vi "TestPVCam_DiskStreaming.vi"(8 "error in":errorcluster, 10 "Exposure time [ms]":T7=25) -> (0 "error out":errorcluster)   [LabVIEW 2023, in "Photometrics Camera.lvlib"]
uses:
  Photometrics Camera.lvlib
  <userlib>/TPM LabVIEW adapter/SDK/Controls/Camera Description.ctl
  <userlib>/TPM LabVIEW adapter/SDK/Controls/Exposure Time.ctl
  <userlib>/TPM LabVIEW adapter/SDK/Controls/Frames To Capture.ctl
  <userlib>/TPM LabVIEW adapter/SDK/Controls/Frames Captured.ctl
  <userlib>/TPM LabVIEW adapter/SDK/Controls/Disk Streaming Options.ctl
  <userlib>/TPM LabVIEW adapter/SDK/Controls/Disk Streaming File Name.ctl
  <userlib>/TPM LabVIEW adapter/SDK/Controls/Disk Streaming File Size.ctl
  <userlib>/TPM LabVIEW adapter/PVCAM/PVCAM.lvclass
  <userlib>/TPM LabVIEW adapter/SDK/Controls/All Params IDs.ctl
  <userlib>/TPM LabVIEW adapter/SDK/Controls/Acquisition Mode.ctl
  <userlib>/TPM LabVIEW adapter/SDK/Controls/Region Index.ctl
  <userlib>/TPM LabVIEW adapter/SDK/Controls/Buffer Size.ctl
  <userlib>/TPM LabVIEW adapter/Camera/Camera.lvclass
panel:
  in  "Disk Streaming Options":T1={"Disk Streaming File Name"="test", "Path"=path "E:/", "File Format"=enum."RAW", "File Size"=1000000000000, "Big TIFF required"=FALSE}
  out "Frames Captured":T4
  out "Image":T5(plugin-control)
  in  "Frames To Capture":T6=1000
  out "Disk Streaming Failed":bool
  out "Disk Streaming Dropped Frames":u64
  out "FPS":dbl
  out "Disk Streaming Queue Count":u32
  out "Camera Description":T8
  out "Number of cameras":u32
  out "Camera 0 Name":string
  out "output array":u16[][](array[numeric])
  in  "STOP":bool
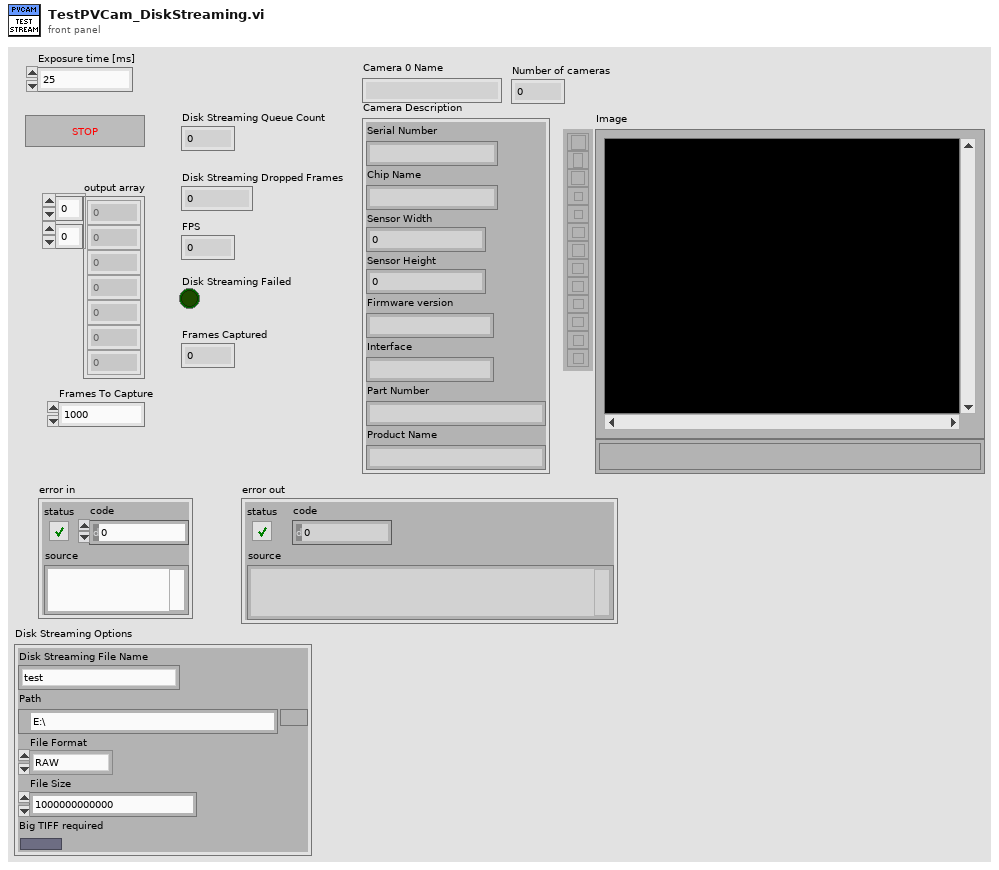
[diagram p1: front panel]
types:
  T1 = typedef "Disk Streaming Options.ctl" = cluster{"Disk Streaming File Name":T2, "Path":path, "File Format":enum32{"RAW", "TIFF"}, "File Size":T3, "Big TIFF required":bool}
  T2 = typedef "Disk Streaming File Name.ctl" = string
  T3 = typedef "Disk Streaming File Size.ctl" = u64
  T4 = typedef "Frames Captured.ctl" = u64
  T5 = typedef "IMAQ Image.ctl" = refnum<image>
  T6 = typedef "Frames To Capture.ctl" = u32
  T7 = typedef "Exposure Time.ctl" = u32
  T8 = typedef "Camera Description.ctl" = cluster{"Serial Number":string, "Chip Name":string, "Sensor Width":u32, "Sensor Height":u32, "Firmware version":string, "Interface":string, "Part Number":string, "Product Name":string}
  T9 = typedef "Buffer Size.ctl" = u32
  T10 = typedef "Region Index.ctl" = i32
  T11 = typedef "Acquisition Mode.ctl" = enum16{"Sequence", "Live"}
  T12 = typedef "All Params IDs.ctl" = i32
  T13 = typedef "Camera Regions.ctl" = T14[]
  T14 = typedef "Region.ctl" = cluster{"Origin X":u16, "Origin Y":u16, "Width":u16, "Height":u16}
  T15 = typedef "Acquisition Status.ctl" = enum32{"Idle", "Starting", "Acquiring", "Stopping"}
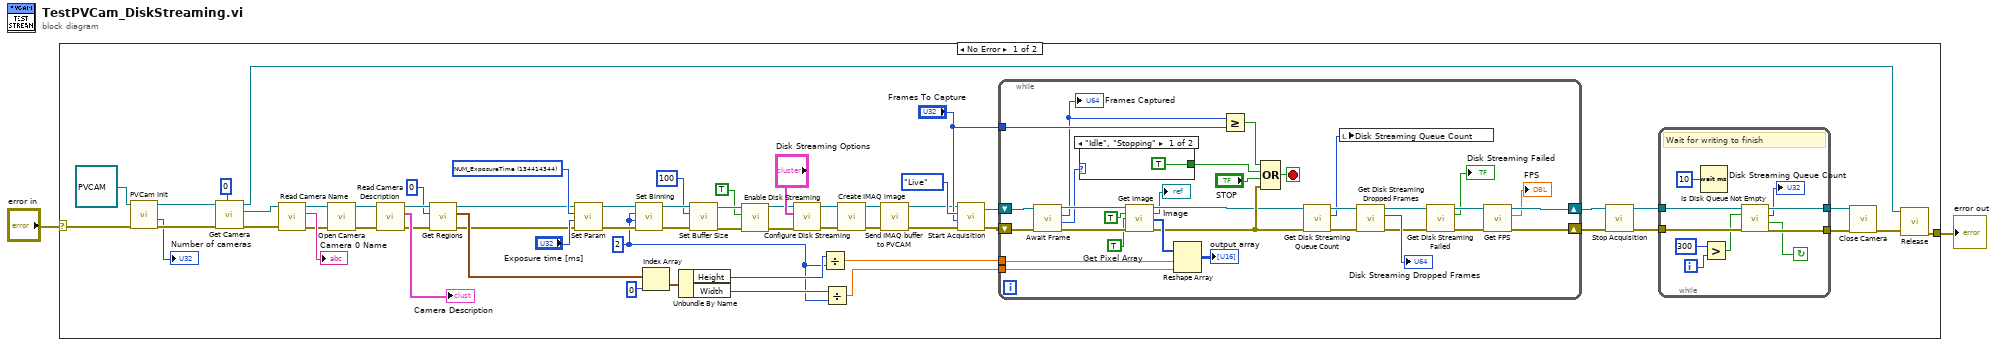
[diagram p0: block diagram]
diagram:
  n1 = case shown="No Error" "error in" {
    selector: "error in" -> [w30 w105]
    tunnel: [w41 w105] -> w2
    frame No Error {
      w8 = u16 2 ("Binning X")
      w47 = T12 134414344 items=["BOOL_BofEofClr"=184745991, "BOOL_CentroidsEnabled"=184746154, "BOOL_CircBuffer"=184746283, "BOOL_FrameCapable"=184680957, "BOOL_GainMultEnable"=184680989, "BOOL_MetadataEnabled"=184746152, "BOOL_MetadataResetTimestamp"=184746160, "BOOL_ScanDirectionReset"=184746236, "BOOL_SmartStreamModeEnabled"=184681148, "ENUM_BinningPar"=151191718, "ENUM_BinningSer"=151191717, "ENUM_BofEofEnable"=151191557, "ENUM_CamInterfaceMode"=150994955, "ENUM_CamInterfaceType"=150994954, "ENUM_CentroidsBgCount"=151191726, "ENUM_CentroidsMode"=151191725, "ENUM_ClearMode"=151126539, "ENUM_ColorMode"=151126520, "ENUM_CoolingMode"=151126230, "ENUM_ExpRes"=151191554, "ENUM_ExposeOutMode"=151126576, "ENUM_ExposureMode"=151126551, "ENUM_FanSpeedSetpoint"=151126726, "ENUM_FrameFlip"=151126273, "ENUM_FrameRotate"=151126272, "ENUM_ImageCompression"=151126265, "ENUM_ImageFormat"=151126264, "ENUM_IoDirection"=151126545, "ENUM_IoType"=151126544, "ENUM_MppCapable"=151126240, "ENUM_PMode"=151126540, "ENUM_ReadoutPort"=151126263, "ENUM_ScanDirection"=151191803, "ENUM_ScanMode"=151191802, "ENUM_ShtrOpenMode"=151126537, "ENUM_ShtrStatus"=151126538, "ENUM_TrigTabSignal"=151191732, "NUM_ActualGain"=100794912, "NUM_AdcOffset"=16908483, "NUM_BitDepth"=16908799, "NUM_BofEofCount"=117637126, "NUM_CamFwVersion"=100794900, "NUM_CentroidsCount"=100860076, "NUM_CentroidsRadius"=100860075, "NUM_CentroidsThreshold"=117637295, "NUM_ClearCycles"=100794465, "NUM_ClearingTime"=268566708, "NUM_DdInfoLength"=16777217, "NUM_DdRetries"=100663299, "NUM_DdTimeout"=100663300, "NUM_DdVersion"=100663298, "NUM_ExpResIndex"=100859908, "NUM_ExpTime"=100859905, "NUM_ExposureTime"=134414344, "NUM_FrameBufferSize"=134414636, "NUM_FwellCapacity"=117572090, "NUM_GainIndex"=16908800, "NUM_GainMultFactor"=100794905, "NUM_IoAddr"=100794895, "NUM_IoBitDepth"=100794899, "NUM_IoState"=67240466, "NUM_LastMuxedSignal"=84082869, "NUM_ParSize"=100794425, "NUM_PciFwVersion"=100794902, "NUM_PixParDist"=100794868, "NUM_PixParSize"=100794431, "NUM_PixSerDist"=100794869, "NUM_PixSerSize"=100794430, "NUM_PixTime"=100794884, "NUM_PostTriggerDelay"=268566709, "NUM_Postmask"=100794422, "NUM_Postscan"=100794424, "NUM_PreTriggerDelay"=268566710, "NUM_PreampDelay"=100794870, "NUM_PreampOffControl"=117572091, "NUM_Premask"=100794421, "NUM_Prescan"=100794423, "NUM_ReadoutTime"=67240115, "NUM_RoiCount"=100860073, "NUM_SP_PpIndex"=16908831, "NUM_SP_PpParamIndex"=16908833, "NUM_ScanLineDelay"=100860157, "NUM_ScanLineTime"=268632318, "NUM_ScanWidth"=100860159, "NUM_SerSize"=100794426, "NUM_ShtrCloseDelay"=100794887, "NUM_ShtrOpenDelay"=100794888, "NUM_SmartStreamMode"=100795069, "NUM_SpdtabIndex"=16908801, "NUM_SummingWell"=184680953, "NUM_Temp"=16908813, "NUM_TempSetpoint"=16908814, "PP_PpFeatId"=100794917, "PP_PpParam"=117572131, "PP_PpParamId"=100794918, "PP_ReadNoise"=100794916, "SS_SmartStreamDlyParams"=235012799, "SS_SmartStreamModeExpParams"=235012798, "STR_CamSystemsInfo"=218235416, "STR_CameraPartNumber"=218235013, "STR_ChipName"=218235009, "STR_DdInfo"=218103813, "STR_GainName"=218235394, "STR_HeadSerNumAlpha"=218235413, "STR_PpFeatName"=218235422, "STR_PpParamName"=218235426, "STR_ProductName"=218235012, "STR_SystemName"=218235010, "STR_VendorName"=218235011] ("PVCAM Param IDs")
      n2 = call <userlib>:"PVCam Init.vi"("error in (no error)"=w30, "PVCAM In"=refnum<class "PVCAM.lvclass"> refnum ("PVCAM.lvclass")) -> ("error out"=w58:errorcluster, "Number of cameras"=→"Number of cameras":u32, "PVCAM Out"=w60:refnum<class "PVCAM.lvclass">)  [unwired: 6 in, 1 out]
      n3 = call <userlib>:"Get Camera.vi"("Camera Index"=u32 0 ("Camera Index (0)"), "error in (no error)"=w58, "PVCAM In"=w60) -> ("error out"=w55:errorcluster, "Camera.lvclass"=w57:refnum<class "Camera.lvclass">, "PVCAM Out"=w61:refnum<class "PVCAM.lvclass">)  [unwired: 6 in]
      n4 = call <userlib>:"Read Camera Name.vi"("error in (no error)"=w55, "Camera in"=w57) -> ("error out"=w53:errorcluster, "Camera Name"=→"Camera 0 Name":string, "Camera out"=w54:refnum<class "Camera.lvclass">)  [unwired: 7 in]
      n5 = call <userlib>:"Open Camera.vi"("error in (no error)"=w53, "Camera in"=w54) -> ("error out"=w50:errorcluster, "Camera out"=w49:refnum<class "Camera.lvclass">)  [unwired: 8 in]
      n6 = call-dynamic "Read Camera Description.vi"("error in (no error)"=w50, "Camera in"=w49) -> ("error out"=w37:errorcluster, "Camera Description"=→"Camera Description":T8, "Camera out"=w38:refnum<class "Camera.lvclass">)  [unwired: 7 in]
      n7 = call <userlib>:"Get Regions.vi"("error in (no error)"=w37, "Region Index"=T10 0, "Camera in"=w38) -> ("error out"=w19:errorcluster, "Camera Regions"=w33:T13, "Camera out"=w20:refnum<class "Camera.lvclass">)  [unwired: 6 in]
      n8 = call <userlib>:"Set Param.vi"("error in (no error)"=w19, "Parameter value"="Exposure time [ms]", "PVCAM Param IDs"=w47, "Camera In"=w20) -> ("error out"=w45:errorcluster, "Camera Out"=w44:refnum<class "Camera.lvclass">)  [unwired: 6 in]
      n9 = call <userlib>:"Set Binning.vi"("error in (no error)"=w45, "Binning Y"=w8, "Binning X"=w8, "Camera in"=w44) -> ("error out"=w24:errorcluster, "Camera out"=w23:refnum<class "Camera.lvclass">)  [unwired: 6 in]
      n10 = Index Array(array=w33, index=0) -> (element=w35:T14)
      n11 = Unbundle By Name(w35) -> ("Height"=w11:u16, "Width"=w9:u16)
      n12 = call <userlib>:"Set Buffer Size.vi"("error in (no error)"=w24, "Buffer Size Frames"=T9 100, "Camera in"=w23) -> ("error out"=w6:errorcluster, "Camera out"=w7:refnum<class "Camera.lvclass">)  [unwired: 7 in]
      n13 = call <userlib>:"Enable Disk Streaming.vi"("error in (no error)"=w6, "Enable/Disable streaming"=TRUE, "Camera in"=w7) -> ("error out"=w5:errorcluster, "Camera out"=w4:refnum<class "Camera.lvclass">)  [unwired: 7 in]
      n14 = call <userlib>:"Configure Disk Streaming.vi"("error in (no error)"=w5, "Disk Streaming Options"="Disk Streaming Options", "Camera in"=w4) -> ("error out"=w17:errorcluster, "Camera out"=w13:refnum<class "Camera.lvclass">)  [unwired: 7 in]
      n15 = Divide(x=w11, y=w8) -> (x/y=w12:dbl)
      n16 = Divide(x=w9, y=w8) -> (x/y=w10:dbl)
      n17 = call <userlib>:"Create IMAQ image.vi"("error in (no error)"=w17, "Camera in"=w13) -> ("error out"=w18:errorcluster, "Camera out"=w14:refnum<class "Camera.lvclass">)  [unwired: 8 in]
      n18 = call <userlib>:"Send IMAQ buffer to PVCAM.vi"("error in (no error)"=w18, "Camera in"=w14) -> ("error out"=w16:errorcluster, "Camera out"=w15:refnum<class "Camera.lvclass">)  [unwired: 8 in]
      n19 = call <userlib>:"Start Acquisition.vi"("error in (no error)"=w16, "Frames To Capture"="Frames To Capture", "Acquisition Mode"=Acquisition_Mode."Live", "Camera in"=w15) -> ("error out"=w40:errorcluster, "Camera out"=w39:refnum<class "Camera.lvclass">)  [unwired: 6 in]
      n20 = while {
        shift-right: [w88] -> w31
        shift-left: w39 -> [w102]
        shift-right: [w89] -> w32
        shift-left: w40 -> [w103]
        tunnel: w12 -> [w96]
        tunnel: w10 -> [w95]
        tunnel: "Frames To Capture" -> [w74]
        stop <- w92 stop-if-true
        w98 = TRUE  # Get Pixel Array
        n21 = call <userlib>:"Await Frame.vi"("error in (no error)"=w103, "Camera in"=w102) -> ("error out"=w101:errorcluster, "Acquisition Status"=w93:T15, "Frames Captured"=w73:T4, "Camera out"=w100:refnum<class "Camera.lvclass">)  [unwired: 6 in]
        "Frames Captured" <- w73
        n22 = case shown="\"Idle\", \"Stopping\"" w93 {
          tunnel: [TRUE ("value") _] -> w91
          frame "Idle", "Stopping" {
          }
          frame Default {
          }
        }
        n23 = call <userlib>:"Get Image.vi"("Camera in"=w100, "Get Image (T)"=TRUE, "Get Pixel Array (F)"=w98, "error in (no error)"=w101) -> ("Camera out"=w83:refnum<class "Camera.lvclass">, "IMAQ image"=→"Image":T5, "Pixels UNS16"=w97:u16[], "error out"=w86:errorcluster)  [unwired: 6 in, 2 out]
        n24 = Reshape Array(w97, w96, w95) -> (→"output array":u16[][])
        n25 = Greater Or Equal?(x=w73, y=w74) -> (x >= y?=w72:bool)
        n26 = Compound Arithmetic op=OR(w72, w91, "STOP", w86) -> (w92:bool)
        n27 = call <userlib>:"Get Disk Streaming Queue Count.vi"("error in (no error)"=w86, "Camera in"=w83) -> ("error out"=w85:errorcluster, "Disk Streaming Queue Count"=w82:u32, "Camera out"=w84:refnum<class "Camera.lvclass">)  [unwired: 7 in]
        n28 = local write "Disk Streaming Queue Count"(w82) -> ()
        n29 = call <userlib>:"Get Disk Streaming Dropped Frames.vi"("error in (no error)"=w85, "Camera in"=w84) -> ("error out"=w80:errorcluster, "Disk Streaming Dropped Frames"=→"Disk Streaming Dropped Frames":u64, "Camera out"=w78:refnum<class "Camera.lvclass">)  [unwired: 7 in]
        n30 = call <userlib>:"Get Disk Streaming Failed.vi"("error in (no error)"=w80, "Camera in"=w78) -> ("error out"=w79:errorcluster, "Disk Streaming Failed"=→"Disk Streaming Failed":bool, "Camera out"=w77:refnum<class "Camera.lvclass">)  [unwired: 7 in]
        n31 = call <userlib>:"Get FPS.vi"("error in (no error)"=w79, "Camera in"=w77) -> ("error out"=w89:errorcluster, "FPS"=→"FPS":dbl, "Camera out"=w88:refnum<class "Camera.lvclass">)  [unwired: 7 in]
      }
      n32 = call <userlib>:"Stop Acquisition.vi"("error in (no error)"=w32, "Camera in"=w31) -> ("error out"=w28:errorcluster, "Camera out"=w27:refnum<class "Camera.lvclass">)  [unwired: 8 in]
      n33 = while {
        tunnel: w28 -> [w71]
        tunnel: w27 -> [w70]
        tunnel: [w69] -> w26
        tunnel: [w64] -> w25
        i -> [w68]
        stop <- w63 continue-if-true
        # "Wait for writing to finish"
        n34 = Wait (ms)(milliseconds to wait=u32 10) -> ()  [unwired: 1 out]
        n35 = Greater?(x=300, y=w68) -> (0:w67:bool)
        n36 = call <userlib>:"Is Disk Queue Not Empty.vi"("error in (no error)"=w71, "Abort Flushing To Disk"=w67, "Camera in"=w70) -> ("error out"=w64:errorcluster, "Disk Queue Not Empty"=w63:bool, "Disk Streaming Queue Count"=→"Disk Streaming Queue Count":u32, "Camera out"=w69:refnum<class "Camera.lvclass">)  [unwired: 5 in]
      }
      n37 = call <userlib>:"Close Camera.vi"("error in (no error)"=w25, "Camera in"=w26) -> ("error out"=w42:errorcluster)  [unwired: 8 in, 1 out]
      n38 = call <userlib>:"Release.vi"("error in (no error)"=w42, "PVCAM in"=w61) -> ("error out"=w41:errorcluster)  [unwired: 8 in, 1 out]
    }
    frame Error {
    }
  }
  "error out" <- w2
